vi "Periodic Tasks.vi"(8 "error in":errorcluster) -> ()   [LabVIEW 2018]
doc: "This VI runs in parallel to other tasks. It can contain as many user-defined periodic loops as you need. These can carry out PID or other sorts of timed response."
uses:
  Robot Global Data.vi
  <vilib>/Rock Robotics/Network Tables/NT Write Numeric Array.vi
  <vilib>/Rock Robotics/Network Tables/NT Write Boolean Array.vi
  <vilib>/Rock Robotics/Network Tables/NT Read Number.vi
  <vilib>/Rock Robotics/WPI/DriverStation/WPI_DriverStationRobotMode2.ctl
  <vilib>/Rock Robotics/Network Tables/NT Write String.vi
  <vilib>/Rock Robotics/Network Tables/NT Write Number.vi
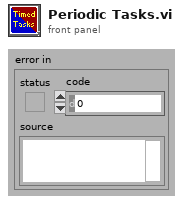
[diagram p1: front panel]
types:
  T1 = typedef "WPI_GyroDevRef.ctl" = cluster{"DevStatus":errorcluster, "Analog Channel":T2, "Gain (VoltsPerDegree/Second)":dbl, "Gyro Type":enum16{"Analog", "XRS450"}, "Handle":i32, "SPI Bus":T3, "Device Found":bool, "Sample Rate":dbl, "Calibrate On Open":bool, "Offset":dbl}
  T2 = typedef "FPGA_AIChannel.ctl" = enum8{"AI 0", "AI 1", "AI 2", "AI 3", "AI MXP 0", "AI MXP 1", "AI MXP 2", "AI MXP 3", "Invalid"}
  T3 = typedef "spi_bus.ctl" = enum16{"SPI On-Board, CS0", "SPI On-Board, CS1", "SPI On-Board, CS2", "SPI On-Board, CS3", "SPI MXP", "Invalid"}
  T4 = typedef "WPI_JoystickDevRef.ctl" = cluster{"Device":T5}
  T5 = typedef "WPI_JoystickDeviceEnum.ctl" = enum16{"USB 0", "USB 1", "USB 2", "USB 3", "USB 4", "USB 5"}
  T6 = typedef "WPI_RobotDriveDevRef.ctl" = cluster{"DevStatus":errorcluster, "Motors[]":T7[], "Square Inputs":bool, "Max Output":dbl}
  T7 = typedef "WPI_MotorControlDeviceRef.ctl" = cluster{"DeviceStatus":errorcluster, "Type":T8, "PWM":cluster{"PWM Channel":T9, "DeadBand":T10}, "CAN":cluster{"Device Number":u8, "SetOutput VI Ref":variant, "GetOutput VI Ref":variant, "Enable VI Ref":variant, "Disable VI Ref":variant, "Data":variant}, "Invert":bool, "DIO PWM":cluster{"PWM \"Enable\" Channel":T9, "DIOChannel":T11, "PWM Rate":dbl}}
  T8 = typedef "WPI_MotorControlType.ctl" = enum16{"PWM", "CAN", "DIO PWM"}
  T9 = typedef "FPGA_DIOPWMChannel.ctl" = enum8{"PWM 0", "PWM 1", "PWM 2", "PWM 3", "PWM 4", "PWM 5", "PWM 6", "PWM 7", "PWM 8", "PWM 9", "PWM MXP 0", "PWM MXP 1", "PWM MXP 2", "PWM MXP 3", "PWM MXP 4", "PWM MXP 5", "PWM MXP 6", "PWM MXP 7", "PWM MXP 8", "PWM MXP 9", "Invalid"}
  T10 = typedef "WPI_PWMDeadband.ctl" = cluster{"Name":string, "maxPositivePwm":i32, "minPositivePwm":i32, "centerPwm":i32, "maxNegativePwm":i32, "minNegativePwm":i32, "angularRange":u16}
  T11 = typedef "FPGA_DIOChannel.ctl" = enum8{"DIO 0", "DIO 1", "DIO 2", "DIO 3", "DIO 4", "DIO 5", "DIO 6", "DIO 7", "DIO 8", "DIO 9", "DIO MXP 0", "DIO MXP 1", "DIO MXP 2", "DIO MXP 3", "DIO MXP 4", "DIO MXP 5", "DIO MXP 6", "DIO MXP 7", "DIO MXP 8", "DIO MXP 9", "DIO MXP 10", "DIO MXP 11", "DIO MXP 12", "DIO MXP 13", "DIO MXP 14", "DIO MXP 15", "SPI Port CS1", "SPI Port CS2", "SPI Port CS3", "SPI Port MISO", "SPI Port MOSI", "Invalid"}
  T12 = cluster{"JoystickDevRef":T4, "JoystickDevRef":T4, "RobotDriveDevRef":T6, "GyroDevRef":T1}
  T13 = typedef "WPI_DriverStationRobotMode2.ctl" = enum16{"Autonomous Disabled", "Autonomous Enabled", "Teleop Disabled", "Teleop Enabled", "Disconnected", "Finish", "Test Disabled", "Test Enabled", "Emergency Stopped"}
  T14 = typedef "WPI_DriverStationPositionInfo.ctl" = enum16{"1", "2", "3"}
  T15 = typedef "WPI_DriverStationAllianceInfo.ctl" = enum16{"Red", "Blue", "Invalid"}
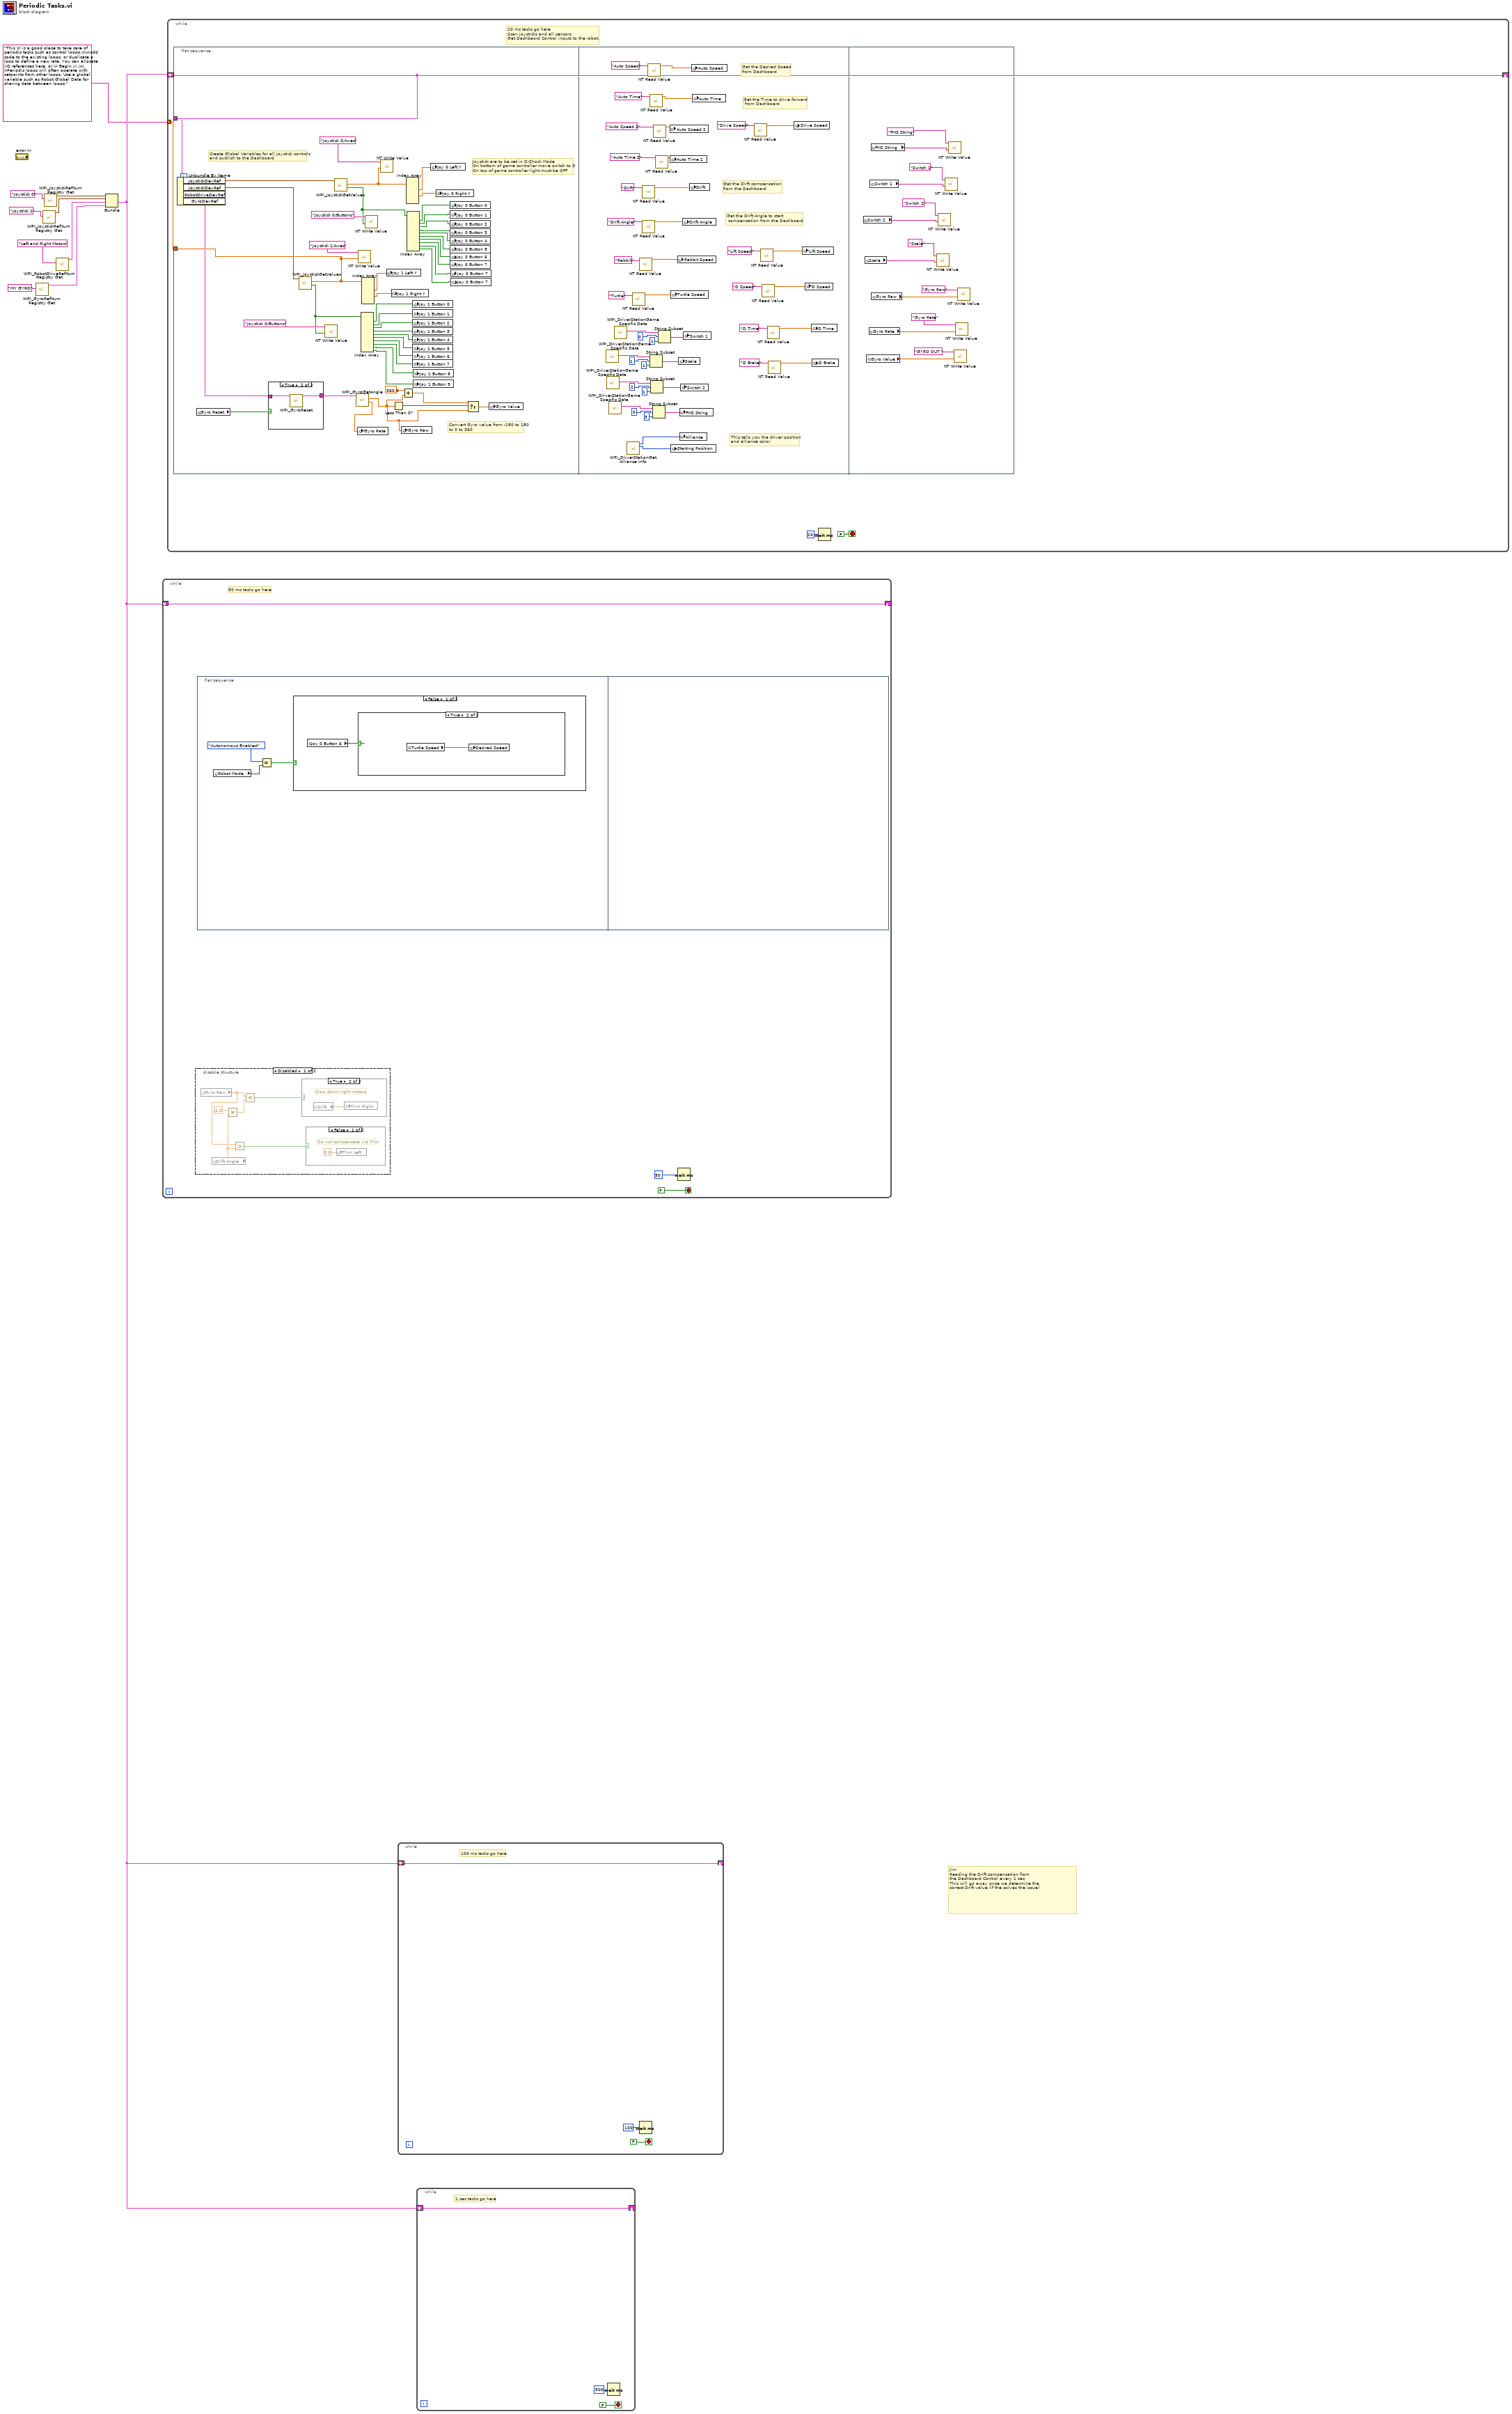
[diagram p0: block diagram]
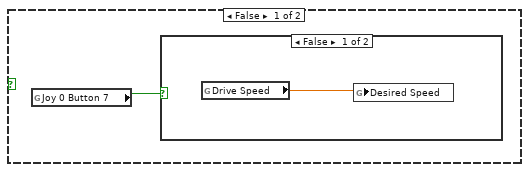
[diagram p2: hidden frame]
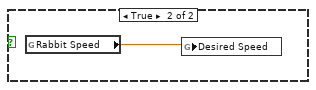
[diagram p3: hidden frame]
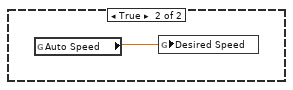
[diagram p4: hidden frame]
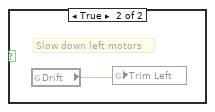
[diagram p5: hidden frame]
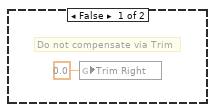
[diagram p6: hidden frame]
diagram:
  # "Jim\nReading the Drift compensation from\nthe Dashboard Control every 1 sec\nThis will go away once we determine the\ncorrect Drift value (if the solves the issue)"
  n1 = call <vilib>:"WPI_GyroRefNum Registry Get.vi"("refnum name"="MY GYRO") -> ("GyroDevRef"=w3:T1)  [unwired: 9 in, 1 out]
  n2 = call <vilib>:"WPI_JoystickRefNum Registry Get.vi"("refnum name"="Joystick 1") -> ("JoystickDevRef"=w4:T4)  [unwired: 9 in, 1 out]
  n3 = call <vilib>:"WPI_JoystickRefNum Registry Get.vi"("refnum name"="Joystick 0") -> ("JoystickDevRef"=w7:T4)  [unwired: 9 in, 1 out]
  n4 = call <vilib>:"WPI_RobotDriveRefNum Registry Get.vi"("refnum name"="Left and Right Motors") -> ("RobotDriveDevRef"=w6:T6)  [unwired: 1 in, 9 out]
  n5 = Bundle("JoystickDevRef"=w7, "JoystickDevRef"=w4, "RobotDriveDevRef"=w6, "GyroDevRef"=w3) -> (w2:T12)  [unwired: 1 out]
  n6 = while {
    shift-right: [w11] -> _
    shift-left: w2 -> [w11]
    stop <- FALSE stop-if-true
    # "50 ms tasks go here"
    n7 = disable-structure shown="Disabled" {
      frame Disabled {
        n8 = global read "Robot Global Data.vi" "Gyro Raw"() -> (w26:dbl)
        n9 = global read "Robot Global Data.vi" "Drift Angle"() -> (w28:dbl)
        n10 = Multiply(x=-1.0, y=w28) -> (x*y=w27:dbl)
        n11 = Greater?(x=w26, y=w28) -> (0:w23:bool)
        n12 = Less?(x=w26, y=w27) -> (x < y?=w24:bool)
        n13 = case shown="True" w24 {
          frame False {
            # "Do not compensate via Trim"
            n14 = global write "Robot Global Data.vi" "Trim Right"(0.0 ("Trim Right")) -> ()
          }
          frame True {
            # "Slow down right motors"
            n15 = global read "Robot Global Data.vi" "Drift"() -> (w32:dbl)
            n16 = global write "Robot Global Data.vi" "Trim Right"(w32) -> ()
          }
        }
        n17 = case shown="False" w23 {
          frame False {
            # "Do not compensate via Trim"
            n18 = global write "Robot Global Data.vi" "Trim Left"(0.0 ("Trim Right")) -> ()
          }
          frame True {
            # "Slow down left motors"
            n19 = global read "Robot Global Data.vi" "Drift"() -> (w30:dbl)
            n20 = global write "Robot Global Data.vi" "Trim Left"(w30) -> ()
          }
        }
      }
      frame Enabled {
      }
    }
    n21 = flat-sequence {
      frame #0 {
        n22 = global read "Robot Global Data.vi" "Robot Mode"() -> (w15:T13)
        n23 = Equal?(x=WPI_DriverStationRobotMode2."Autonomous Enabled", y=w15) -> (x = y?=w16:bool)
        n24 = case shown="False" w16 {
          frame False {
            n25 = global read "Robot Global Data.vi" "Joy 0 Button 6"() -> (w17:bool)
            n26 = case shown="True" w17 {
              frame False {
                n27 = global read "Robot Global Data.vi" "Joy 0 Button 7"() -> (w18:bool)
                n28 = case shown="False" w18 {
                  frame False {
                    n29 = global read "Robot Global Data.vi" "Drive Speed"() -> (w19:dbl)
                    n30 = global write "Robot Global Data.vi" "Desired Speed"(w19) -> ()
                  }
                  frame True {
                    n31 = global read "Robot Global Data.vi" "Rabbit Speed"() -> (w20:dbl)
                    n32 = global write "Robot Global Data.vi" "Desired Speed"(w20) -> ()
                  }
                }
              }
              frame True {
                n33 = global read "Robot Global Data.vi" "Turtle Speed"() -> (w21:dbl)
                n34 = global write "Robot Global Data.vi" "Desired Speed"(w21) -> ()
              }
            }
          }
          frame True {
            n35 = global read "Robot Global Data.vi" "Auto Speed"() -> (w22:dbl)
            n36 = global write "Robot Global Data.vi" "Desired Speed"(w22) -> ()
          }
        }
      }
      frame #1 {
      }
    }
    n37 = Wait (ms)(milliseconds to wait=u32 50) -> ()  [unwired: 1 out]
  }
  n38 = while {
    shift-right: [w34] -> _
    shift-left: w2 -> [w34]
    tunnel: "This VI is a good place to take care of periodic tasks such as control loops.\n\nAdd code to the existing loops, or duplicate a loop to define a new rate. You can allocate I/O references here, or in Begin.vi.\n\nPeriodic loops will often operate with setpoints from other loops. Use a global variable such as Robot Global Data for sharing data between loops." -> [w33]
    stop <- FALSE stop-if-true
    # "20 ms tasks go here\nScan joysticks and all sensors\nGet Dashbaord Control inputs to the robot."
    n39 = flat-sequence {
      tunnel: w34 -> [w74]
      tunnel: [w37] -> w33
      frame #0 {
        # "Create Global Variables for all Joystick controls\nand publish to the Dashboard"
        # "Convert Gyro value from -180 to 180\nto 0 to 360"
        # "Joystick are to be set in D-Shock Mode\nOn bottom of game controller move switch to D\nOn top of game controller light must be OFF"
        n40 = Unbundle By Name(w74) -> ("JoystickDevRef"=w73:T4, "JoystickDevRef"=w58:T4, "GyroDevRef"=w43:T1)  [unwired: 1 out]
        n41 = global read "Robot Global Data.vi" "Gyro Reset"() -> (w42:bool)
        n42 = case shown="True" w42 {
          tunnel: [w81 w83] -> w44
          tunnel: w43 -> [w81 w82]
          frame False {
          }
          frame True {
            n43 = call <vilib>:"WPI_GyroReset.vi"("GyroDevRef"=w82) -> ("GyroDevRef"=w83:T1)  [unwired: 9 in, 1 out]
          }
        }
        n44 = call <vilib>:"WPI_JoystickGetValues.vi"("JoystickDevRef"=w58) -> ("Buttons"=w53:bool[], "Axes"=w37:dbl[])  [unwired: 6 in, 3 out]
        n45 = call-poly <vilib>:"NT Write Value.vi"("Boolean Array"=w53, "Name"="Joystick 0/Buttons") -> ()  [unwired: 9 in, 1 out]
        n46 = call <vilib>:"WPI_JoystickGetValues.vi"("JoystickDevRef"=w73) -> ("Buttons"=w67:bool[], "Axes"=w70:dbl[])  [unwired: 6 in, 3 out]
        n47 = call <vilib>:"WPI_GyroGetAngle.vi"("GyroDevRef"=w44) -> ("Angular Rate"=w76:dbl, "Angle"=w75:dbl)  [unwired: 6 in, 3 out]
        n48 = global write "Robot Global Data.vi" "Gyro Rate"(w76) -> ()
        n49 = call-poly <vilib>:"NT Write Value.vi"("Numeric Array"=w37, "Name"="Joystick 1/Axes") -> ()  [unwired: 9 in, 1 out]
        n50 = Index Array(array=w53) -> (element #1=w52:bool, element #2=w51:bool, element #3=w50:bool, element #4=w49:bool, element #5=w48:bool, element #6=w47:bool, element #7=w46:bool, element #8=w45:bool, element #9=w41:bool, element #10=w40:bool)  [unwired: 10 in]
        n51 = Index Array(array=w37) -> (element #2=w55:dbl, element #4=w56:dbl)  [unwired: 6 in, 4 out]
        n52 = call-poly <vilib>:"NT Write Value.vi"("Boolean Array"=w67, "Name"="Joystick 0/Buttons") -> ()  [unwired: 9 in, 1 out]
        n53 = call-poly <vilib>:"NT Write Value.vi"("Numeric Array"=w70, "Name"="Joystick 0/Axes") -> ()  [unwired: 9 in, 1 out]
        n54 = global write "Robot Global Data.vi" "Joy 1 Left Y"(w55) -> ()
        n55 = global write "Robot Global Data.vi" "Joy 1 Right Y"(w56) -> ()
        n56 = Less Than 0?(x=w75) -> (x < 0?=w79:bool)
        n57 = global write "Robot Global Data.vi" "Gyro Raw"(w75) -> ()
        n58 = Add(x=360.0 ("y"), y=w75) -> (x+y=w78:dbl)
        n59 = Index Array(array=w70) -> (element #2=w69:dbl, element #4=w68:dbl)  [unwired: 6 in, 4 out]
        n60 = Index Array(array=w67) -> (element #1=w66:bool, element #2=w65:bool, element #3=w64:bool, element #4=w63:bool, element #5=w62:bool, element #6=w61:bool, element #7=w60:bool, element #8=w59:bool, element #9=w39:bool, element #10=w38:bool)  [unwired: 10 in]
        n61 = global write "Robot Global Data.vi" "Joy 1 Button 0"(w52) -> ()
        n62 = global write "Robot Global Data.vi" "Joy 1 Button 1"(w51) -> ()
        n63 = global write "Robot Global Data.vi" "Joy 1 Button 2"(w50) -> ()
        n64 = global write "Robot Global Data.vi" "Joy 1 Button 3"(w49) -> ()
        n65 = global write "Robot Global Data.vi" "Joy 1 Button 4"(w48) -> ()
        n66 = global write "Robot Global Data.vi" "Joy 1 Button 5"(w47) -> ()
        n67 = global write "Robot Global Data.vi" "Joy 1 Button 6"(w46) -> ()
        n68 = global write "Robot Global Data.vi" "Joy 1 Button 7"(w45) -> ()
        n69 = global write "Robot Global Data.vi" "Joy 1 Button 8"(w41) -> ()
        n70 = global write "Robot Global Data.vi" "Joy 1 Button 9"(w40) -> ()
        n71 = global write "Robot Global Data.vi" "Joy 0 Left Y"(w69) -> ()
        n72 = global write "Robot Global Data.vi" "Joy 0 Right Y"(w68) -> ()
        n73 = global write "Robot Global Data.vi" "Joy 0 Button 0"(w66) -> ()
        n74 = global write "Robot Global Data.vi" "Joy 0 Button 1"(w65) -> ()
        n75 = global write "Robot Global Data.vi" "Joy 0 Button 2"(w64) -> ()
        n76 = global write "Robot Global Data.vi" "Joy 0 Button 3"(w63) -> ()
        n77 = global write "Robot Global Data.vi" "Joy 0 Button 4"(w62) -> ()
        n78 = global write "Robot Global Data.vi" "Joy 0 Button 5"(w61) -> ()
        n79 = global write "Robot Global Data.vi" "Joy 0 Button 6"(w60) -> ()
        n80 = global write "Robot Global Data.vi" "Joy 0 Button 7"(w59) -> ()
        n81 = global write "Robot Global Data.vi" "Joy 0 Button 7"(w39) -> ()
        n82 = global write "Robot Global Data.vi" "Joy 0 Button 7"(w38) -> ()
        n83 = Select(t=w78, s=w79, f=w75) -> (s? t:f=w80:dbl)
        n84 = global write "Robot Global Data.vi" "Gyro Value"(w80) -> ()
      }
      frame #1 {
        # "Get the Drift Angle to start\n compensation from the Dashboard"
        # "This tells you the driver position\nand alliance color"
        # "Get the Time to drive forward\n from Dashboard"
        # "Get the Desired Speed \nfrom Dashboard"
        # "Get the Drift compensation\nfrom the Dashboard"
        n85 = call <vilib>:"WPI_DriverStationGame Specific Data.vi"() -> ("Game Specific Data"=w114:string)  [unwired: 11 in]
        n86 = call <vilib>:"WPI_DriverStationGame Specific Data.vi"() -> ("Game Specific Data"=w115:string)  [unwired: 11 in]
        n87 = call <vilib>:"WPI_DriverStationGame Specific Data.vi"() -> ("Game Specific Data"=w122:string)  [unwired: 11 in]
        n88 = call <vilib>:"WPI_DriverStationGame Specific Data.vi"() -> ("Game Specific Data"=w113:string)  [unwired: 11 in]
        n89 = call <vilib>:"WPI_DriverStationGet Alliance Info.vi"() -> ("Position"=w119:T14, "Alliance"=w120:T15)  [unwired: 10 out]
        n90 = call-poly <vilib>:"NT Read Value.vi"("Name"="Turtle") -> ("Numeric"=w127:dbl)  [unwired: 9 in, 1 out]
        n91 = call-poly <vilib>:"NT Read Value.vi"("Name"="Rabbit") -> ("Numeric"=w124:dbl)  [unwired: 9 in, 1 out]
        n92 = call-poly <vilib>:"NT Read Value.vi"("Name"="Drift") -> ("Numeric"=w110:dbl)  [unwired: 9 in, 1 out]
        n93 = call-poly <vilib>:"NT Read Value.vi"("Name"="Drift Angle") -> ("Numeric"=w123:dbl)  [unwired: 9 in, 1 out]
        n94 = call-poly <vilib>:"NT Read Value.vi"("Name"="Auto Speed") -> ("Numeric"=w111:dbl)  [unwired: 9 in, 1 out]
        n95 = call-poly <vilib>:"NT Read Value.vi"("Name"="Auto Time") -> ("Numeric"=w112:dbl)  [unwired: 9 in, 1 out]
        n96 = String Subset(string=w114, offset (0)=1, length (rest)=1 ("length (rest)")) -> (substring=w117:string)
        n97 = String Subset(string=w115, offset (0)=2, length (rest)=1 ("length (rest)")) -> (substring=w118:string)
        n98 = String Subset(string=w122, offset (0)=0, length (rest)=3 ("length (rest)")) -> (substring=w121:string)
        n99 = call-poly <vilib>:"NT Read Value.vi"("Name"="Auto Speed 2") -> ("Numeric"=w126:dbl)  [unwired: 9 in, 1 out]
        n100 = call-poly <vilib>:"NT Read Value.vi"("Name"="Auto Time 2") -> ("Numeric"=w125:dbl)  [unwired: 9 in, 1 out]
        n101 = String Subset(string=w113, offset (0)=0, length (rest)=1 ("length (rest)")) -> (substring=w116:string)
        n102 = global write "Robot Global Data.vi" "Auto Speed 2"(w126) -> ()
        n103 = global write "Robot Global Data.vi" "Auto Time 2"(w125) -> ()
        n104 = global write "Robot Global Data.vi" "Starting Position"(w119) -> ()
        n105 = global write "Robot Global Data.vi" "Turtle Speed"(w127) -> ()
        n106 = global write "Robot Global Data.vi" "Rabbit Speed"(w124) -> ()
        n107 = global write "Robot Global Data.vi" "Scale"(w117) -> ()
        n108 = global write "Robot Global Data.vi" "FMS String"(w121) -> ()
        n109 = global write "Robot Global Data.vi" "Alliance"(w120) -> ()
        n110 = global write "Robot Global Data.vi" "Switch 2"(w118) -> ()
        n111 = global write "Robot Global Data.vi" "Drift Angle"(w123) -> ()
        n112 = global write "Robot Global Data.vi" "Switch 1"(w116) -> ()
        n113 = global write "Robot Global Data.vi" "Drift"(w110) -> ()
        n114 = global write "Robot Global Data.vi" "Auto Speed"(w111) -> ()
        n115 = global write "Robot Global Data.vi" "Auto Time"(w112) -> ()
        n116 = call-poly <vilib>:"NT Read Value.vi"("Name"="Drive Speed") -> ("Numeric"=w91:dbl)  [unwired: 9 in, 1 out]
        n117 = call-poly <vilib>:"NT Read Value.vi"("Name"="Lift Speed") -> ("Numeric"=w93:dbl)  [unwired: 9 in, 1 out]
        n118 = call-poly <vilib>:"NT Read Value.vi"("Name"="D Speed") -> ("Numeric"=w88:dbl)  [unwired: 9 in, 1 out]
        n119 = call-poly <vilib>:"NT Read Value.vi"("Name"="D Time") -> ("Numeric"=w87:dbl)  [unwired: 9 in, 1 out]
        n120 = call-poly <vilib>:"NT Read Value.vi"("Name"="D Brake") -> ("Numeric"=w84:dbl)  [unwired: 9 in, 1 out]
        n121 = global write "Robot Global Data.vi" "Drive Speed"(w91) -> ()
        n122 = global write "Robot Global Data.vi" "Lift Speed"(w93) -> ()
        n123 = global write "Robot Global Data.vi" "D Speed"(w88) -> ()
        n124 = global write "Robot Global Data.vi" "D Time"(w87) -> ()
        n125 = global write "Robot Global Data.vi" "D Brake"(w84) -> ()
      }
      frame #2 {
        n126 = global read "Robot Global Data.vi" "Switch 2"() -> (w138:string)
        n127 = global read "Robot Global Data.vi" "Scale"() -> (w135:string)
        n128 = global read "Robot Global Data.vi" "Gyro Value"() -> (w133:dbl)
        n129 = global read "Robot Global Data.vi" "Gyro Rate"() -> (w129:dbl)
        n130 = global read "Robot Global Data.vi" "Switch 1"() -> (w139:string)
        n131 = global read "Robot Global Data.vi" "FMS String"() -> (w141:string)
        n132 = global read "Robot Global Data.vi" "Gyro Raw"() -> (w132:dbl)
        n133 = call-poly <vilib>:"NT Write Value.vi"("String"=w135, "Name"="Scale") -> ()  [unwired: 9 in, 1 out]
        n134 = call-poly <vilib>:"NT Write Value.vi"("String"=w138, "Name"="Switch 2") -> ()  [unwired: 9 in, 1 out]
        n135 = call-poly <vilib>:"NT Write Value.vi"("String"=w139, "Name"="Switch 1") -> ()  [unwired: 9 in, 1 out]
        n136 = call-poly <vilib>:"NT Write Value.vi"("String"=w141, "Name"="FMS String") -> ()  [unwired: 9 in, 1 out]
        n137 = call-poly <vilib>:"NT Write Value.vi"("Numeric"=w133, "Name"="GYRO OUT ") -> ()  [unwired: 9 in, 1 out]
        n138 = call-poly <vilib>:"NT Write Value.vi"("Numeric"=w129, "Name"="Gyro Rate") -> ()  [unwired: 9 in, 1 out]
        n139 = call-poly <vilib>:"NT Write Value.vi"("Numeric"=w132, "Name"="Gyro Raw") -> ()  [unwired: 9 in, 1 out]
      }
    }
    n140 = Wait (ms)(milliseconds to wait=u32 20) -> ()  [unwired: 1 out]
  }
  n141 = while {
    shift-right: [w142] -> _
    shift-left: w2 -> [w142]
    stop <- FALSE stop-if-true
    # "100 ms tasks go here"
    n142 = Wait (ms)(milliseconds to wait=u32 100) -> ()  [unwired: 1 out]
  }
  n143 = while {
    shift-right: [w145] -> _
    shift-left: w2 -> [w145]
    stop <- FALSE stop-if-true
    # "1 sec tasks go here"
    n144 = Wait (ms)(milliseconds to wait=u32 500) -> ()  [unwired: 1 out]
  }
